vi "Event and Sensor Selector 3.1.vi"(8 "error in":errorcluster, 10 "Starting State":T3, 11 "Data Cluster In":T1={"Selected File"=path "", "Full Text File"=[], "Data Array"=[], "Times Array"=[], "Sensor Array"=[], "Subset Array"=[], "Smoothness Values"=[], "Sensor Select 1"=refnum, "Sensor Select 2"=refnum, "Sensor Select 3"=refnum, "Sensor Select 4"=refnum, "Start Times"=[], "End Times"=[], "Cursor List"=[{"Name"="Event Marker          ", "Color"=16777200, "Style"=0, "Point Style"=0, "Name Visible"=FALSE, "Allow Drag"=FALSE, "Cursor Mode"=0, "Plot"=0, "Index"=0, "Position"={"X"=4.0, "Y"=1.0}, "X Scale"=0, "Y Scale"=0, "Watch Plots"=[], "Watch All Plots"=FALSE, "Plot Area"=0, "Label Offset"={"X"=-50.0, "Y"=150.0}}, {"Name"="Upper Sensor", "Color"=13816500, "Style"=6, "Point Style"=0, "Name Visible"=FALSE, "Allow Drag"=FALSE, "Cursor Mode"=0, "Plot"=0, "Index"=0, "Position"={"X"=-1.0, "Y"=5.0}, "X Scale"=0, "Y Scale"=0, "Watch Plots"=[], "Watch All Plots"=FALSE, "Plot Area"=0, "Label Offset"={"X"=0.0, "Y"=0.0}}, {"Name"="Lower Sensor", "Color"=13816500, "Style"=6, "Point Style"=0, "Name Visible"=FALSE, "Allow Drag"=FALSE, "Cursor Mode"=0, "Plot"=0, "Index"=0, "Position"={"X"=-1.0, "Y"=30.0}, "X Scale"=0, "Y Scale"=0, "Watch Plots"=[], "Watch All Plots"=FALSE, "Plot Area"=0, "Label Offset"={"X"=0.0, "Y"=0.0}}], "Listbox 1"=refnum, "Listbox 2"=refnum, "Listbox 3"=refnum, "Listbox 4"=refnum, "Labels"=["Why", "is", "this", "still", "not", "built", "into", "Labview?", "This", "is", "shameful."], "Event Array"=[], "Event Names"=[], "Event Times"=[], "Save Plot Button"=refnum, "Sensor Plot Refs"=[], "Selected Event (Title)"="", "Upper Cursor"=0.0, "Lower Cursor"=0.0, "Z Max"=0.0, "Z Min"=0.0}) -> (0 "error out":errorcluster, 3 "Data Cluster Out":T1={"Selected File"=path "", "Full Text File"=[], "Data Array"=[], "Times Array"=[], "Sensor Array"=[], "Subset Array"=[], "Smoothness Values"=[], "Sensor Select 1"=refnum, "Sensor Select 2"=refnum, "Sensor Select 3"=refnum, "Sensor Select 4"=refnum, "Start Times"=[], "End Times"=[], "Cursor List"=[{"Name"="Event Marker          ", "Color"=16777200, "Style"=0, "Point Style"=0, "Name Visible"=FALSE, "Allow Drag"=FALSE, "Cursor Mode"=0, "Plot"=0, "Index"=0, "Position"={"X"=4.0, "Y"=1.0}, "X Scale"=0, "Y Scale"=0, "Watch Plots"=[], "Watch All Plots"=FALSE, "Plot Area"=0, "Label Offset"={"X"=-50.0, "Y"=150.0}}, {"Name"="Upper Sensor", "Color"=13816500, "Style"=6, "Point Style"=0, "Name Visible"=FALSE, "Allow Drag"=FALSE, "Cursor Mode"=0, "Plot"=0, "Index"=0, "Position"={"X"=-1.0, "Y"=5.0}, "X Scale"=0, "Y Scale"=0, "Watch Plots"=[], "Watch All Plots"=FALSE, "Plot Area"=0, "Label Offset"={"X"=0.0, "Y"=0.0}}, {"Name"="Lower Sensor", "Color"=13816500, "Style"=6, "Point Style"=0, "Name Visible"=FALSE, "Allow Drag"=FALSE, "Cursor Mode"=0, "Plot"=0, "Index"=0, "Position"={"X"=-1.0, "Y"=30.0}, "X Scale"=0, "Y Scale"=0, "Watch Plots"=[], "Watch All Plots"=FALSE, "Plot Area"=0, "Label Offset"={"X"=0.0, "Y"=0.0}}], "Listbox 1"=refnum, "Listbox 2"=refnum, "Listbox 3"=refnum, "Listbox 4"=refnum, "Labels"=["Why", "is", "this", "still", "not", "built", "into", "Labview?", "This", "is", "shameful."], "Event Array"=[], "Event Names"=[], "Event Times"=[], "Save Plot Button"=refnum, "Sensor Plot Refs"=[], "Selected Event (Title)"="", "Upper Cursor"=0.0, "Lower Cursor"=0.0, "Z Max"=0.0, "Z Min"=0.0})   [LabVIEW 2020]
uses:
  Controls/Selector Cases.ctl
  Controls/DataCluster.ctl
  <vilib>/Utility/miscctls.llb/LVCursorListTypeDef.ctl
panel:
  in  "Home Button":bool
  in  "Next Button":bool
  in  "Previous Button":bool
  in  "Event Name":u16(ring)
  in  "Lower Cursor":dbl=-1.0 min=-36.0 max=-1.0 step=1.0
  in  "Upper Cursor":dbl=-1.0 min=-36.0 max=-1.0 step=1.0
  out "Segment Select":dbl[][](graph)
  in  "Listbox 3":i32[](listbox)
  in  "Listbox 2":i32[](listbox)
  in  "Listbox 4":i32[](listbox)
  in  "Listbox":i32[](listbox)
  out "Sensor Plot 2":dynamicdata(graph)
  out "Sensor Plot 1":dynamicdata(graph)
  out "Sensor Plot 4":dynamicdata(graph)
  out "Sensor Plot 3":dynamicdata(graph)
  # "Velopharynx"
  # "Tongue Base"
  # "Hypopharynx"
  # "Click here after selecting an event and sensors."
  # "UES"
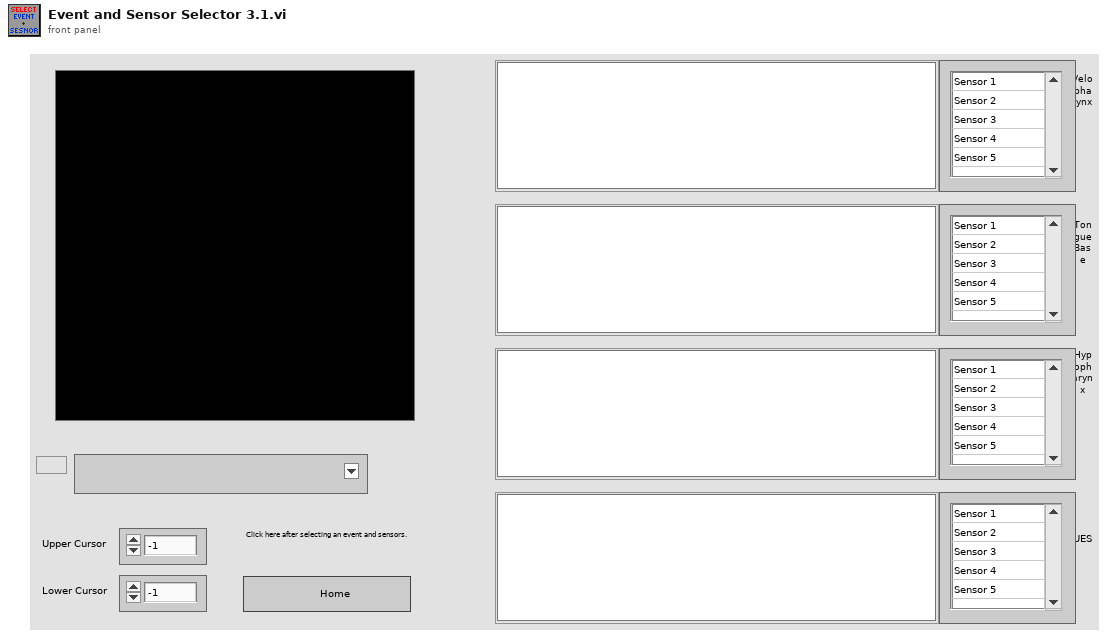
[diagram p1: front panel]
types:
  T1 = typedef "DataCluster.ctl" = cluster{"Selected File":path, "Full Text File":string[][], "Data Array":dbl[][], "Times Array":dbl[], "Sensor Array":dbl[], "Subset Array":dbl[][], "Smoothness Values":dbl[], "Sensor Select 1":refnum<vi>, "Sensor Select 2":refnum<vi>, "Sensor Select 3":refnum<vi>, "Sensor Select 4":refnum<vi>, "Start Times":dbl[], "End Times":dbl[], "Cursor List":T2, "Listbox 1":refnum<vi>, "Listbox 2":refnum<vi>, "Listbox 3":refnum<vi>, "Listbox 4":refnum<vi>, "Labels":string[], "Event Array":dbl[][], "Event Names":string[], "Event Times":dbl[], "Save Plot Button":refnum<vi>, "Sensor Plot Refs":refnum<vi>[], "Selected Event (Title)":string, "Upper Cursor":dbl, "Lower Cursor":dbl, "Z Max":dbl, "Z Min":dbl}
  T2 = typedef "LVCursorListTypeDef.ctl" = cluster{"Name":string, "Color":u32, "Style":u8, "Point Style":u8, "Name Visible":bool, "Allow Drag":bool, "Cursor Mode":u32, "Plot":i32, "Index":i32, "Position":cluster{"X":dbl, "Y":dbl}, "X Scale":u32, "Y Scale":u32, "Watch Plots":i32[], "Watch All Plots":bool, "Plot Area":i32, "Label Offset":cluster{"X":dbl, "Y":dbl}}[]
  T3 = typedef "Selector Cases.ctl" = enum16{"Initialize", "Wait", "Open", "Find Segment", "Update Sensor Plots", "Analyze", "Save", "Exit"}
  T4 = enum16{"None", "On Hover", "On Key Focus", "On Hover or Key Focus"}
  T5 = cluster{"Cursor List[0]":cluster{"Name":string, "Color":u32, "Style":u8, "Point Style":u8, "Name Visible":bool, "Allow Drag":bool, "Cursor Mode":u32, "Plot":i32, "Index":i32, "Position":cluster{"X":dbl, "Y":dbl}, "X Scale":u32, "Y Scale":u32, "Watch Plots":i32[], "Watch All Plots":bool, "Plot Area":i32, "Label Offset":cluster{"X":dbl, "Y":dbl}}, "Cursor List[1]":cluster{"Name":string, "Color":u32, "Style":u8, "Point Style":u8, "Name Visible":bool, "Allow Drag":bool, "Cursor Mode":u32, "Plot":i32, "Index":i32, "Position":cluster{"X":dbl, "Y":dbl}, "X Scale":u32, "Y Scale":u32, "Watch Plots":i32[], "Watch All Plots":bool, "Plot Area":i32, "Label Offset":cluster{"X":dbl, "Y":dbl}}, "Cursor List[2]":cluster{"Name":string, "Color":u32, "Style":u8, "Point Style":u8, "Name Visible":bool, "Allow Drag":bool, "Cursor Mode":u32, "Plot":i32, "Index":i32, "Position":cluster{"X":dbl, "Y":dbl}, "X Scale":u32, "Y Scale":u32, "Watch Plots":i32[], "Watch All Plots":bool, "Plot Area":i32, "Label Offset":cluster{"X":dbl, "Y":dbl}}, "Cursor List[3]":cluster{"Name":string, "Color":u32, "Style":u8, "Point Style":u8, "Name Visible":bool, "Allow Drag":bool, "Cursor Mode":u32, "Plot":i32, "Index":i32, "Position":cluster{"X":dbl, "Y":dbl}, "X Scale":u32, "Y Scale":u32, "Watch Plots":i32[], "Watch All Plots":bool, "Plot Area":i32, "Label Offset":cluster{"X":dbl, "Y":dbl}}, "Cursor List[4]":cluster{"Name":string, "Color":u32, "Style":u8, "Point Style":u8, "Name Visible":bool, "Allow Drag":bool, "Cursor Mode":u32, "Plot":i32, "Index":i32, "Position":cluster{"X":dbl, "Y":dbl}, "X Scale":u32, "Y Scale":u32, "Watch Plots":i32[], "Watch All Plots":bool, "Plot Area":i32, "Label Offset":cluster{"X":dbl, "Y":dbl}}, "Cursor List[5]":cluster{"Name":string, "Color":u32, "Style":u8, "Point Style":u8, "Name Visible":bool, "Allow Drag":bool, "Cursor Mode":u32, "Plot":i32, "Index":i32, "Position":cluster{"X":dbl, "Y":dbl}, "X Scale":u32, "Y Scale":u32, "Watch Plots":i32[], "Watch All Plots":bool, "Plot Area":i32, "Label Offset":cluster{"X":dbl, "Y":dbl}}, "Cursor List[6]":cluster{"Name":string, "Color":u32, "Style":u8, "Point Style":u8, "Name Visible":bool, "Allow Drag":bool, "Cursor Mode":u32, "Plot":i32, "Index":i32, "Position":cluster{"X":dbl, "Y":dbl}, "X Scale":u32, "Y Scale":u32, "Watch Plots":i32[], "Watch All Plots":bool, "Plot Area":i32, "Label Offset":cluster{"X":dbl, "Y":dbl}}, "Cursor List[7]":cluster{"Name":string, "Color":u32, "Style":u8, "Point Style":u8, "Name Visible":bool, "Allow Drag":bool, "Cursor Mode":u32, "Plot":i32, "Index":i32, "Position":cluster{"X":dbl, "Y":dbl}, "X Scale":u32, "Y Scale":u32, "Watch Plots":i32[], "Watch All Plots":bool, "Plot Area":i32, "Label Offset":cluster{"X":dbl, "Y":dbl}}, "Cursor List[8]":cluster{"Name":string, "Color":u32, "Style":u8, "Point Style":u8, "Name Visible":bool, "Allow Drag":bool, "Cursor Mode":u32, "Plot":i32, "Index":i32, "Position":cluster{"X":dbl, "Y":dbl}, "X Scale":u32, "Y Scale":u32, "Watch Plots":i32[], "Watch All Plots":bool, "Plot Area":i32, "Label Offset":cluster{"X":dbl, "Y":dbl}}}
  T6 = cluster{"Name":string, "Color":u32, "Style":u8, "Point Style":u8, "Name Visible":bool, "Allow Drag":bool, "Cursor Mode":u32, "Plot":i32, "Index":i32, "Position":cluster{"X":dbl, "Y":dbl}, "X Scale":u32, "Y Scale":u32, "Watch Plots":i32[], "Watch All Plots":bool, "Plot Area":i32, "Label Offset":cluster{"X":dbl, "Y":dbl}}[]
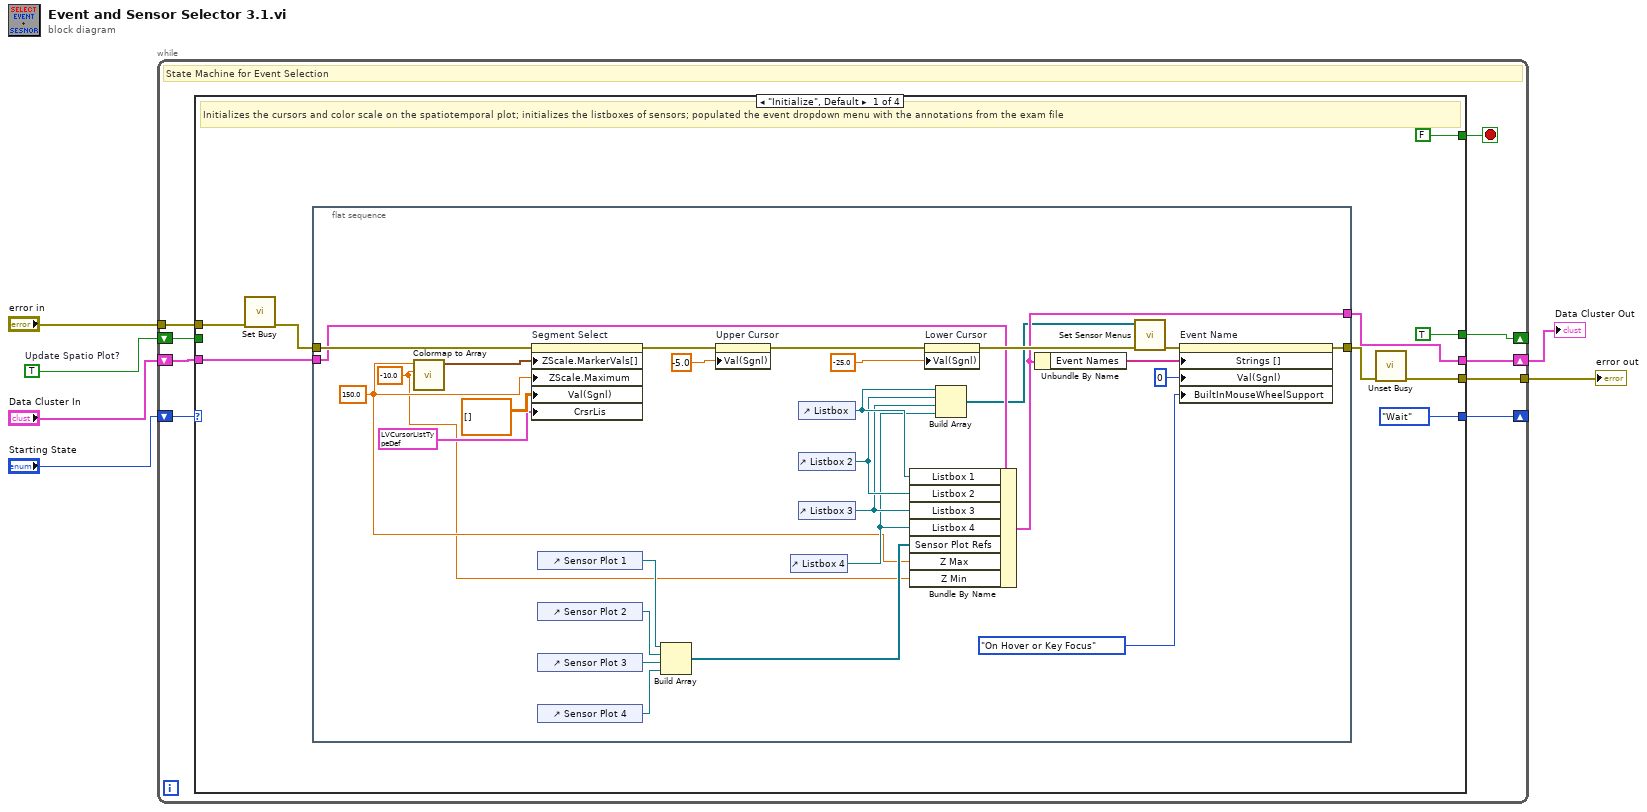
[diagram p0: block diagram]
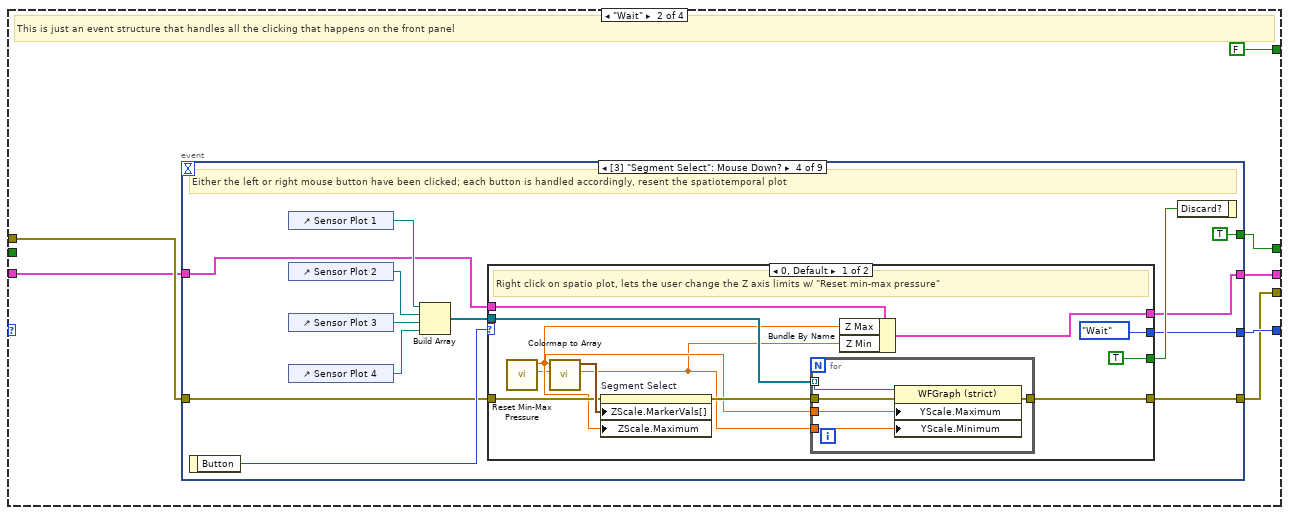
[diagram p2: hidden frame]
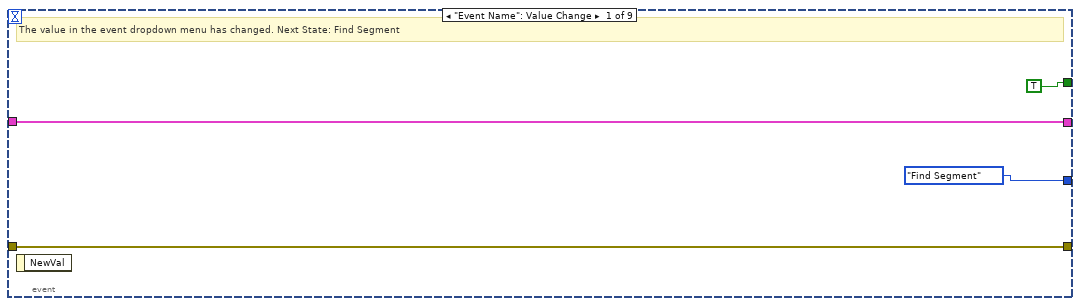
[diagram p3: hidden frame]
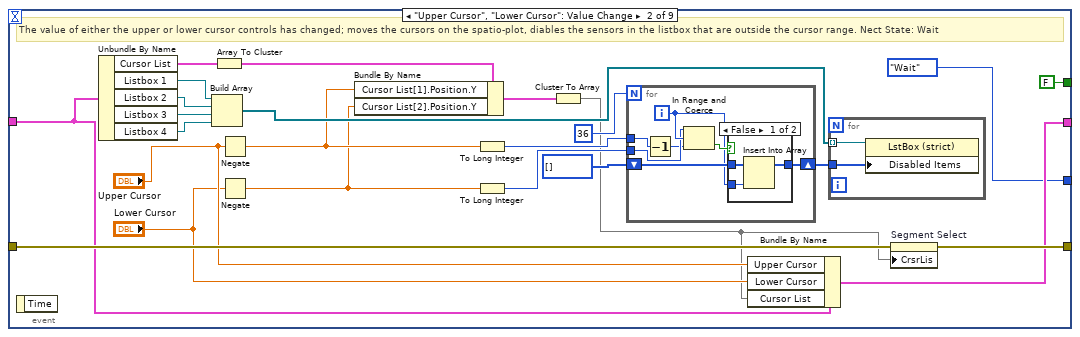
[diagram p4: hidden frame]
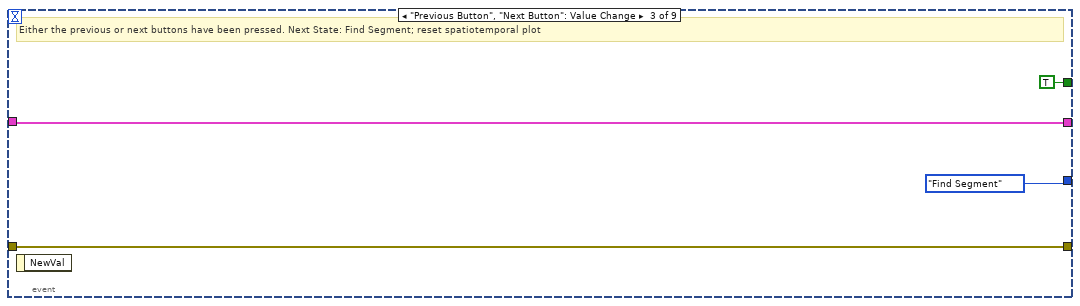
[diagram p6: hidden frame]
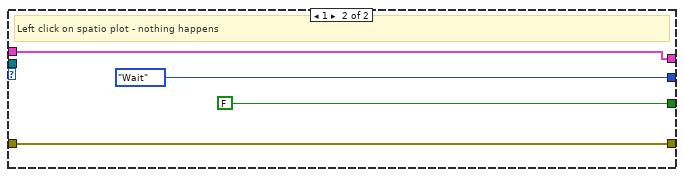
[diagram p7: hidden frame]
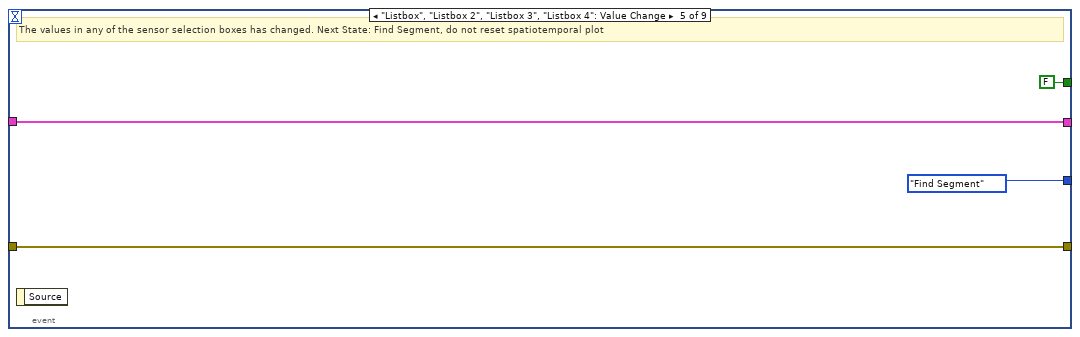
[diagram p8: hidden frame]
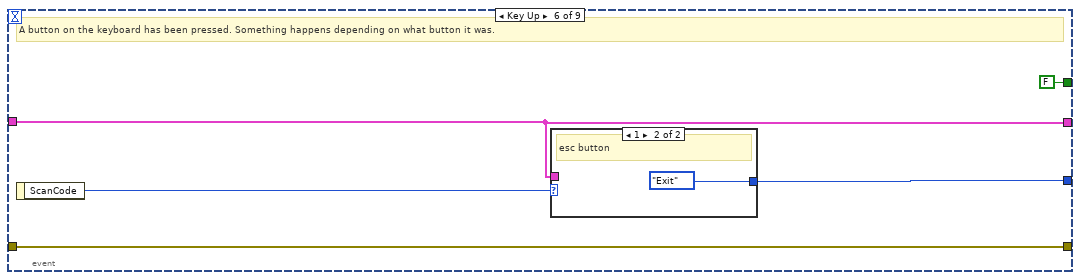
[diagram p9: hidden frame]
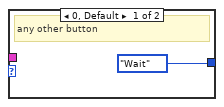
[diagram p10: hidden frame]
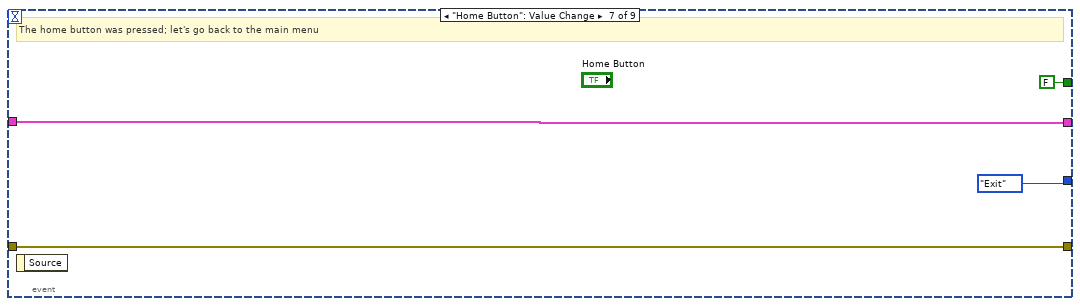
[diagram p11: hidden frame]
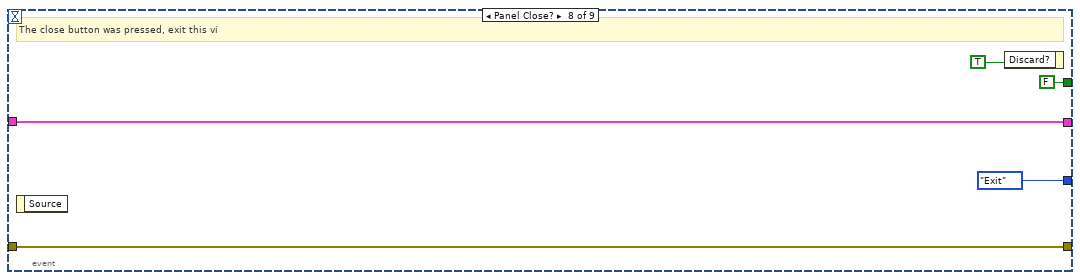
[diagram p12: hidden frame]
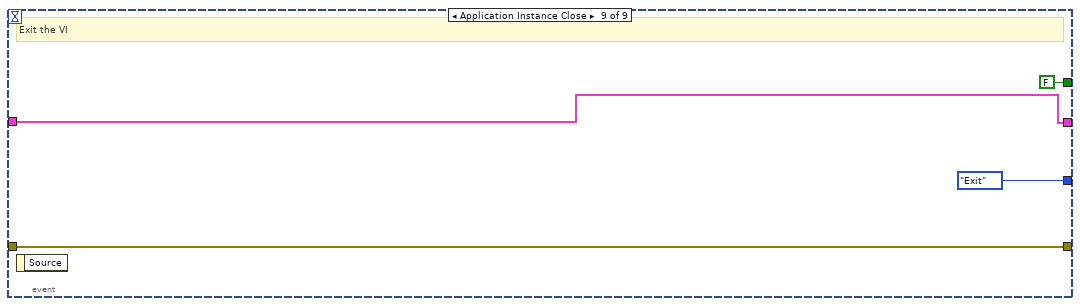
[diagram p13: hidden frame]
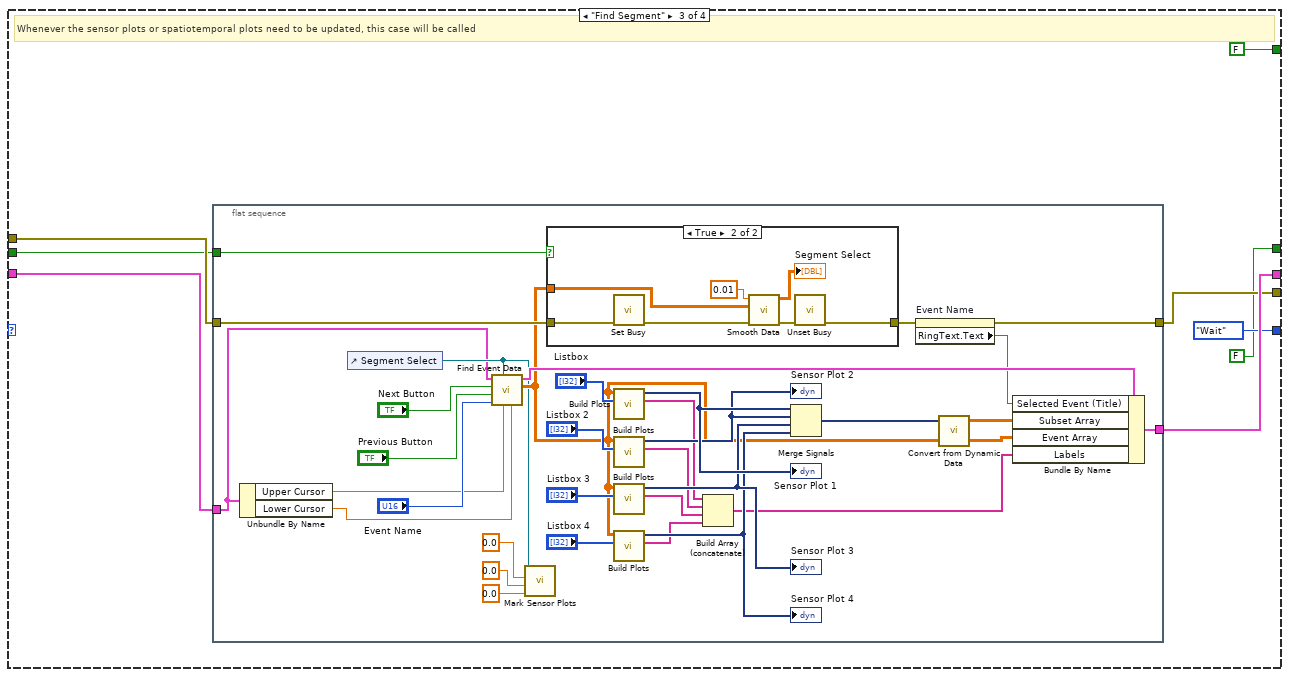
[diagram p14: hidden frame]
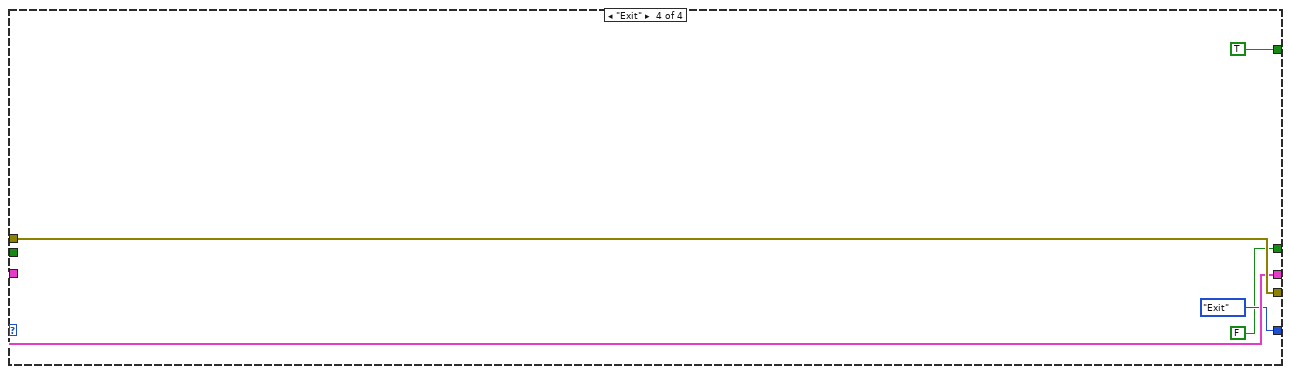
[diagram p16: hidden frame]
diagram:
  w1 = TRUE  # Update Spatio Plot?
  n1 = while {
    shift-right: [w13] -> _
    shift-left: "Starting State" -> [w15]
    shift-right: [w9] -> w2
    shift-left: "Data Cluster In" -> [w12]
    tunnel: "error in" -> [w11]
    tunnel: [w10] -> w5
    shift-right: [w8] -> _
    shift-left: w1 -> [w7]
    stop <- w14 stop-if-true
    # "State Machine for Event Selection"
    n2 = case shown="\"Initialize\", Default" w15 {
      tunnel: [FALSE FALSE FALSE TRUE] -> w14
      tunnel: [Selector_Cases."Wait" ("Starting State 2") w58 Selector_Cases."Wait" ("Starting State") Selector_Cases."Exit" ("Starting State")] -> w13
      tunnel: w12 -> [w23 w55 w167 w213]
      tunnel: [w18 w54 w168 w213] -> w9
      tunnel: w11 -> [w21 w57 w165 w214]
      tunnel: [w19 w56 w164 w214] -> w10
      tunnel: [TRUE w53 FALSE FALSE] -> w8
      tunnel: w7 -> [_ _ w163 _]
      frame "Initialize", Default {
        # "Initializes the cursors and color scale on the spatiotemporal plot; initializes the listboxes of sensors; populated the event dropdown menu with the annotations from the exam file"
        n3 = call <vilib>:"Set Busy.vi"("error in (no error)"=w21) -> ("error out"=w22:errorcluster)  [unwired: 9 in, 1 out]
        n4 = flat-sequence {
          tunnel: w23 -> [w30]
          tunnel: [w32] -> w18
          tunnel: w22 -> [w52]
          tunnel: [w51] -> w20
          frame #0 {
            w26 = -10.0 ("Min Pressure")
            w27 = 150.0 ("Max Pressure")
            n5 = call "Colormap to Array.vi"("Min Pressure"=w26, "Max Pressure"=w27) -> ("Z Scale.Marker Values[]"=w49:cluster{dbl, u32}[])  [unwired: 9 in]
            n6 = property on="Segment Select" class="IntGraph (strict)"(error in=w52, "ZScale.MarkerVals[]"=w49, "ZScale.Maximum"=w27, "Val(Sgnl)"=dbl[][] [] ("Value (Signaling)"), "CrsrLis"=T2 [{"Name"="Event Marker          ", "Color"=16777200, "Style"=0, "Point Style"=0, "Name Visible"=FALSE, "Allow Drag"=FALSE, "Cursor Mode"=0, "Plot"=0, "Index"=0, "Position"={"X"=4.0, "Y"=0.0}, "X Scale"=0, "Y Scale"=0, "Watch Plots"=[], "Watch All Plots"=FALSE, "Plot Area"=0, "Label Offset"={"X"=-50.0, "Y"=150.0}}, {"Name"="Upper Sensor", "Color"=13816500, "Style"=6, "Point Style"=0, "Name Visible"=FALSE, "Allow Drag"=FALSE, "Cursor Mode"=0, "Plot"=0, "Index"=0, "Position"={"X"=-1.0, "Y"=5.0}, "X Scale"=0, "Y Scale"=0, "Watch Plots"=[], "Watch All Plots"=FALSE, "Plot Area"=0, "Label Offset"={"X"=0.0, "Y"=0.0}}, {"Name"="Lower Sensor", "Color"=13816500, "Style"=6, "Point Style"=0, "Name Visible"=FALSE, "Allow Drag"=FALSE, "Cursor Mode"=0, "Plot"=0, "Index"=0, "Position"={"X"=-1.0, "Y"=30.0}, "X Scale"=0, "Y Scale"=0, "Watch Plots"=[], "Watch All Plots"=FALSE, "Plot Area"=0, "Label Offset"={"X"=0.0, "Y"=0.0}}] ("Cursor List")) -> (error out=w42:errorcluster)  [unwired: 1 in, 1 out]
            n7 = control-ref of="Sensor Plot 1"() -> (w37:refnum<vi>)
            n8 = control-ref of="Sensor Plot 2"() -> (w36:refnum<vi>)
            n9 = control-ref of="Sensor Plot 3"() -> (w39:refnum<vi>)
            n10 = control-ref of="Sensor Plot 4"() -> (w38:refnum<vi>)
            n11 = Build Array(w37, w36, w39, w38) -> (w35:refnum<vi>[])
            n12 = property on="Upper Cursor" class="DigNum (strict)"(error in=w42, "Val(Sgnl)"=-5.0 ("Value (Signaling)")) -> (error out=w41:errorcluster)  [unwired: 1 in, 1 out]
            n13 = control-ref of="Listbox 4"() -> (w43:refnum<vi>)
            n14 = control-ref of="Listbox"() -> (w46:refnum<vi>)
            n15 = control-ref of="Listbox 2"() -> (w45:refnum<vi>)
            n16 = control-ref of="Listbox 3"() -> (w44:refnum<vi>)
            n17 = Bundle By Name(cluster=w30, "Listbox 1"=w46, "Listbox 2"=w45, "Listbox 3"=w44, "Listbox 4"=w43, "Sensor Plot Refs"=w35, "Z Max"=w27, "Z Min"=w26) -> (w32:T1)
            n18 = property on="Lower Cursor" class="DigNum (strict)"(error in=w41, "Val(Sgnl)"=-25.0 ("Value (Signaling)")) -> (error out=w40:errorcluster)  [unwired: 1 in, 1 out]
            n19 = Build Array(w46, w45, w44, w43) -> (w25:refnum<vi>[])
            n20 = Unbundle By Name(w32) -> ("Event Names"=w31:string[])
            n21 = call "Set Sensor Menus.vi"("Error In"=w40, "ListBox Refs"=w25) -> ("Error Out"=w34:errorcluster)  [unwired: 9 in]
            n22 = property on="Event Name" class="Ring (strict)"(error in=w34, "Strings []"=w31, "Val(Sgnl)"=u16 0 ("Value (Signaling)"), "BuiltInMouseWheelSupport"=T4."On Hover or Key Focus" ("Built-In Mouse Wheel Support")) -> (error out=w51:errorcluster)  [unwired: 1 in, 1 out]
          }
        }
        n23 = call <vilib>:"Unset Busy.vi"("error in (no error)"=w20) -> ("error out"=w19:errorcluster)  [unwired: 10 in]
      }
      frame "Wait" {
        # "This is just an event structure that handles all the clicking that happens on the front panel"
        n24 = event shown="[3] \"Segment Select\": Mouse Down?" {
          selector: _ -> [_ _ _ _ _ _ _ _ _]
          dyn-events: _ -> [_ _ _ _ _ _ _ _ _]
          timeout: _ -> [_ _ _ _ _ _ _ _ _]
          tunnel: [Selector_Cases."Find Segment" ("Starting State") Selector_Cases."Wait" ("Starting State") Selector_Cases."Find Segment" ("Starting State") w113 Selector_Cases."Find Segment" ("Starting State") w146 Selector_Cases."Exit" ("Starting State") Selector_Cases."Exit" ("Starting State") Selector_Cases."Exit" ("Starting State")] -> w58
          tunnel: w55 -> [w62 w69 w103 w107 w141 w143 w152 w156 w160]
          tunnel: w57 -> [w63 w84 w104 w115 w140 w144 w151 w157 w161]
          tunnel: [w63 w83 w104 w116 w140 w144 w151 w157 w161] -> w56
          tunnel: [w62 w70 w103 w106 w141 w143 w152 w156 w160] -> w54
          tunnel: [TRUE FALSE TRUE TRUE FALSE FALSE FALSE FALSE FALSE] -> w53
          event "Event Name": Value Change {
            # "The value in the event dropdown menu has changed. Next State: Find Segment"
            n25 = event-data() -> ()  [unwired: 1 in, 1 out]
          }
          event "Upper Cursor", "Lower Cursor": Value Change {
            # "The value of either the upper or lower cursor controls has changed; moves the cursors on the spatio-plot, diables the sensors in the listbox that are outside the cursor range. Nect State: Wait"
            n26 = event-data() -> ()  [unwired: 1 in, 1 out]
            n27 = Unbundle By Name(w69) -> ("Cursor List"=w87:T2, "Listbox 1"=w82:refnum<vi>, "Listbox 2"=w81:refnum<vi>, "Listbox 3"=w80:refnum<vi>, "Listbox 4"=w79:refnum<vi>)
            n28 = Build Array(w82, w81, w80, w79) -> (w78:refnum<vi>[])
            n29 = Array To Cluster(array=w87) -> (cluster=w86:T5)
            n30 = Negate(x="Upper Cursor") -> (-x=w77:dbl)
            n31 = Negate(x="Lower Cursor") -> (-x=w76:dbl)
            n32 = Bundle By Name(cluster=w86, "Cursor List[1].Position.Y"=w77, "Cursor List[2].Position.Y"=w76) -> (w85:T5)
            n33 = To Long Integer(number=w77) -> (32bit integer=w73:i32)
            n34 = To Long Integer(number=w76) -> (32bit integer=w72:i32)
            n35 = Cluster To Array(cluster=w85) -> (array=w66:T6)
            n36 = for {
              N: 36 -> [_]
              shift-right: [w91] -> w74
              shift-left: i32[] [] ("Disabled Items") -> [w93]
              tunnel: w73 -> [w89]
              tunnel: w72 -> [w90]
              i -> [w92]
              n37 = Decrement(x=w89) -> (x-1=w88:i32)
              n38 = In Range and Coerce(upper limit=w90, x=w92, lower limit=w88) -> (In Range?=w94:bool)  [unwired: 1 out]
              n39 = case shown="False" w94 {
                tunnel: w93 -> [w97 w98]
                tunnel: w92 -> [w96 _]
                tunnel: [w95 w98] -> w91
                frame False {
                  n40 = Insert Into Array(array=w97, new element=w96) -> (w95:i32[])  [unwired: 1 in]
                }
                frame True {
                }
              }
            }
            n41 = Bundle By Name(cluster=w69, "Upper Cursor"="Upper Cursor", "Lower Cursor"="Lower Cursor", "Cursor List"=w66) -> (w70:T1)
            n42 = for {
              tunnel: w78 -> [w100] mode=indexing
              tunnel: w74 -> [w99]
              n43 = property on="Property Node" class="LstBox (strict)"(reference=w100, "Disabled Items"=w99) -> ()  [unwired: 1 in, 2 out]
            }
            n44 = property on="Segment Select" class="IntGraph (strict)"(error in=w84, "CrsrLis"=w66) -> (error out=w83:errorcluster)  [unwired: 1 in, 1 out]
          }
          event "Previous Button", "Next Button": Value Change {
            # "Either the previous or next buttons have been pressed. Next State: Find Segment; reset spatiotemporal plot"
            n45 = event-data() -> ()  [unwired: 1 in, 1 out]
          }
          event "Segment Select": Mouse Down? {
            # "Either the left or right mouse button have been clicked; each button is handled accordingly, resent the spatiotemporal plot"
            n46 = event-data() -> ("Button"=w117:u16)  [unwired: 1 in]
            n47 = control-ref of="Sensor Plot 1"() -> (w112:refnum<vi>)
            n48 = control-ref of="Sensor Plot 2"() -> (w111:refnum<vi>)
            n49 = control-ref of="Sensor Plot 3"() -> (w110:refnum<vi>)
            n50 = control-ref of="Sensor Plot 4"() -> (w108:refnum<vi>)
            n51 = Build Array(w112, w111, w110, w108) -> (w109:refnum<vi>[])
            n52 = case shown="0, Default" w117 {
              tunnel: [w123 w137] -> w116
              tunnel: w115 -> [w126 w137]
              tunnel: [TRUE FALSE] -> w114
              tunnel: [Selector_Cases."Wait" ("Starting State") Selector_Cases."Wait" ("Starting State")] -> w113
              tunnel: w109 -> [w124 _]
              tunnel: w107 -> [w122 w135]
              tunnel: [w121 w135] -> w106
              frame 0, Default {
                # "Right click on spatio plot, lets the user change the Z axis limits w/ \"Reset min-max pressure\""
                n53 = call "Reset Min-Max Pressure.vi"() -> ("Min Pressure Out"=w119:dbl, "Max Pressure Out"=w120:dbl)  [unwired: 10 in]
                n54 = call "Colormap to Array.vi"("Min Pressure"=w119, "Max Pressure"=w120) -> ("Z Scale.Marker Values[]"=w127:cluster{dbl, u32}[])  [unwired: 9 in]
                n55 = property on="Segment Select" class="IntGraph (strict)"(error in=w126, "ZScale.MarkerVals[]"=w127, "ZScale.Maximum"=w120) -> (error out=w125:errorcluster)  [unwired: 1 in, 1 out]
                n56 = for {
                  tunnel: w125 -> [w133]
                  tunnel: w124 -> [w132] mode=indexing
                  tunnel: [w131] -> w123
                  tunnel: w120 -> [w130]
                  tunnel: w119 -> [w129]
                  n57 = property on="Property Node" class="WFGraph (strict)"(reference=w132, error in=w133, "YScale.Maximum"=w130, "YScale.Minimum"=w129) -> (error out=w131:errorcluster)  [unwired: 1 out]
                }
                n58 = Bundle By Name(cluster=w122, "Z Max"=w120, "Z Min"=w119) -> (w121:T1)
              }
              frame 1 {
                # "Left click on spatio plot - nothing happens"
              }
            }
            n59 = event-data("Discard?"=w114) -> ()  [unwired: 1 in, 1 out]
          }
          event "Listbox", "Listbox 2", "Listbox 3", "Listbox 4": Value Change {
            # "The values in any of the sensor selection boxes has changed. Next State: Find Segment, do not reset spatiotemporal plot"
            n60 = event-data() -> ()  [unwired: 1 in, 1 out]
          }
          event Key Up {
            # "A button on the keyboard has been pressed. Something happens depending on what button it was."
            n61 = event-data() -> ("ScanCode"=w145:i16)  [unwired: 1 in]
            n62 = case shown="1" w145 {
              tunnel: [Selector_Cases."Wait" ("Starting State") Selector_Cases."Exit" ("Starting State")] -> w146
              tunnel: w143 -> [_ _]
              frame 0, Default {
                # "any other button"
              }
              frame 1 {
                # "esc button"
              }
            }
          }
          event "Home Button": Value Change {
            # "The home button was pressed; let's go back to the main menu"
            n63 = event-data() -> ()  [unwired: 1 in, 1 out]
          }
          event Panel Close? {
            # "The close button was pressed, exit this vi"
            n64 = event-data() -> ()  [unwired: 1 in, 1 out]
            n65 = event-data("Discard?"=TRUE) -> ()  [unwired: 1 in, 1 out]
          }
          event Application Instance Close {
            # "Exit the VI"
            n66 = event-data() -> ()  [unwired: 1 in, 1 out]
          }
        }
      }
      frame "Find Segment" {
        # "Whenever the sensor plots or spatiotemporal plots need to be updated, this case will be called"
        n67 = flat-sequence {
          tunnel: [w202] -> w168
          tunnel: w167 -> [w175]
          tunnel: [w173] -> w164
          tunnel: w165 -> [w194]
          tunnel: w163 -> [w171]
          frame #0 {
            n68 = Unbundle By Name(w175) -> ("Upper Cursor"=w181:dbl, "Lower Cursor"=w180:dbl)
            n69 = control-ref of="Segment Select"() -> (w185:refnum<vi>)
            n70 = call "Find Event Data.vi"("Lower Sensor"=w180, "Upper Sensor"=w181, "Intensity Plot Ref"=w185, "Event Name"="Event Name", "Backward"="Previous Button", "Forward"="Next Button", "Data Cluster In"=w175) -> ("Event Data Array"=w186:dbl[][], "output cluster"=w197:T1)  [unwired: 3 in]
            n71 = call "Mark Sensor Plots.vi"("Segment Select Ref"=w185, "Segement Start"=0.0, "End"=0.0, "Start"=0.0) -> ()  [unwired: 7 in]
            n72 = case shown="True" w171 {
              tunnel: w194 -> [w203 w204]
              tunnel: w186 -> [_ w209]
              tunnel: [w203 w207] -> w174
              frame False {
              }
              frame True {
                n73 = call <vilib>:"Set Busy.vi"("error in (no error)"=w204) -> ("error out"=w205:errorcluster)  [unwired: 9 in, 1 out]
                n74 = call "Smooth Data.vi"("error in (no error)"=w205, "Data Array"=w209, "dt"=0.01) -> ("error out"=w206:errorcluster, "Resampled Array"=→"Segment Select":dbl[][])  [unwired: 7 in]
                n75 = call <vilib>:"Unset Busy.vi"("error in (no error)"=w206) -> ("error out"=w207:errorcluster)  [unwired: 10 in]
              }
            }
            n76 = call "Build Plots.vi"("Listbox"="Listbox", "Event Data Array in"=w186) -> ("Labels"=w179:string[], "Sensor Plots"=w193:dynamicdata)  [unwired: 8 in]
            "Sensor Plot 1" <- w193
            n77 = call "Build Plots.vi"("Listbox"="Listbox 2", "Event Data Array in"=w186) -> ("Labels"=w178:string[], "Sensor Plots"=w192:dynamicdata)  [unwired: 8 in]
            "Sensor Plot 2" <- w192
            n78 = call "Build Plots.vi"("Listbox"="Listbox 3", "Event Data Array in"=w186) -> ("Labels"=w177:string[], "Sensor Plots"=w191:dynamicdata)  [unwired: 8 in]
            "Sensor Plot 3" <- w191
            n79 = call "Build Plots.vi"("Listbox"="Listbox 4", "Event Data Array in"=w186) -> ("Labels"=w176:string[], "Sensor Plots"=w190:dynamicdata)  [unwired: 8 in]
            "Sensor Plot 4" <- w190
            n80 = Build Array (concatenate)(w179, w178, w177, w176) -> (w170:string[])
            n81 = Merge Signals(w193, w192, w191, w190) -> (w187:dynamicdata)
            n82 = property on="Event Name" class="Ring (strict)"(error in=w174) -> (error out=w173:errorcluster, "RingText.Text"=w172:string)  [unwired: 1 in, 1 out]
            n83 = call "Convert from Dynamic Data"("Dynamic Data Type"=w187) -> ("Array"=w189:dbl[][])  [unwired: 3 in]
            n84 = Bundle By Name(cluster=w197, "Selected Event (Title)"=w172, "Subset Array"=w189, "Event Array"=w186, "Labels"=w170) -> (w202:T1)
          }
        }
      }
      frame "Exit" {
      }
    }
  }
  "error out" <- w5
  "Data Cluster Out" <- w2
